vi "Write Commands.vi"(8 "error in (no error)":errorcluster, 10 "Commands":refnum<class "WriteCommand.lvclass">[](array[class]), 11 "CommandDirector in":refnum<class "CommandDirector.lvclass">) -> (0 "error out":errorcluster, 3 "CommandDirector out":refnum<class "CommandDirector.lvclass">)   [LabVIEW 2023, in "HAF.lvlib" / "CommandDirector.lvclass"]
doc: "Stores a new collection of Commands."
uses:
  CommandDirector.lvclass
  CommandDirector.lvclass/CommandDirector.ctl
  WriteCommand/WriteCommand.lvclass
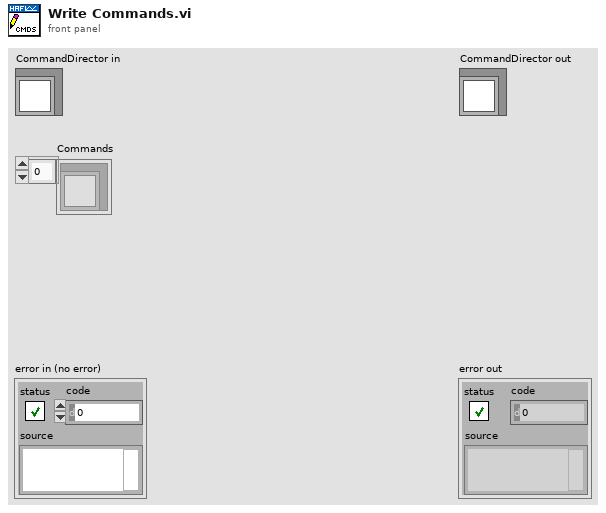
[diagram p1: front panel]
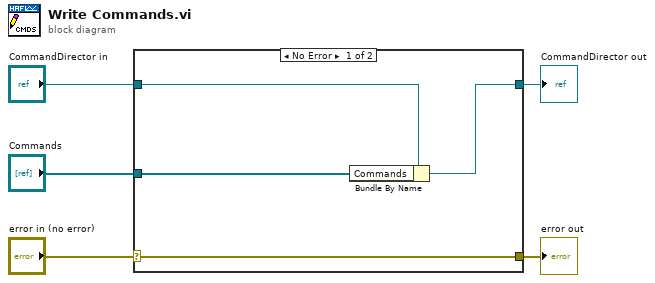
[diagram p0: block diagram]
diagram:
  n1 = case shown="No Error" "error in (no error)" {
    selector: "error in (no error)" -> [w9 w10]
    tunnel: [w9 w10] -> w4
    tunnel: [w7 w11] -> w2
    tunnel: "CommandDirector in" -> [w8 w11]
    tunnel: "Commands" -> [w6 _]
    frame No Error {
      n2 = Bundle By Name(cluster=w8, "Commands"=w6) -> (w7:refnum<class "CommandDirector.lvclass">)
    }
    frame Error {
    }
  }
  "error out" <- w4
  "CommandDirector out" <- w2
